vi "Modules DAQ.vi"(8 "error in (no error)":errorcluster) -> (0 "error out":errorcluster)   [LabVIEW 2020]
uses:
  MOTOR/MOTOR.lvlib
  DMM/PalmSens.lvlib
  Hiden Scanner/Hiden Scanner.lvlib
  MRC/MRC Module.lvlib
  WM Pump/Pump.lvlib
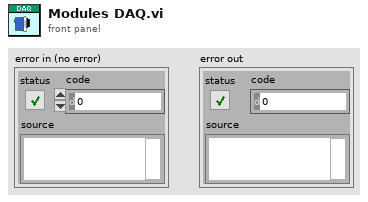
[diagram p1: front panel]
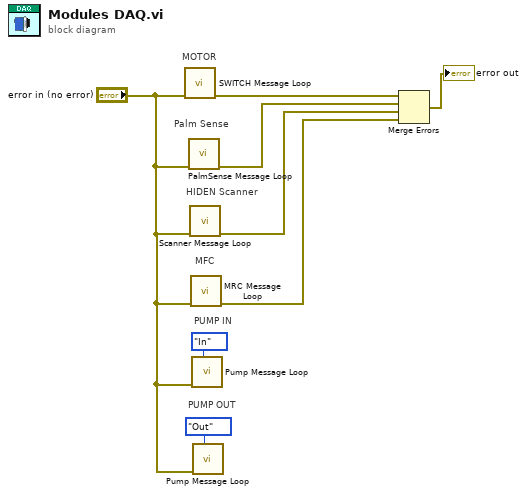
[diagram p0: block diagram]
diagram:
  # "PUMP OUT"
  # "PUMP IN"
  # "MFC"
  # "HIDEN Scanner"
  # "Palm Sense"
  # "MOTOR"
  n1 = call "SWITCH Message Loop.vi"("error in (no error)"="error in (no error)") -> ("error out"=w7:errorcluster)  [unwired: 10 in]
  n2 = call "PalmSense Message Loop.vi"("error in (no error)"="error in (no error)") -> ("error out"=w6:errorcluster)  [unwired: 10 in]
  n3 = call "Scanner Message Loop.vi"("error in (no error)"="error in (no error)") -> ("error out"=w5:errorcluster)  [unwired: 10 in]
  n4 = call "MRC Message Loop.vi"("error in (no error)"="error in (no error)") -> ("error out"=w4:errorcluster)  [unwired: 10 in]
  n5 = call "Pump Message Loop.vi"("Manual Pump Select"=enum32{"In", "Out"}."In", "error in (no error)"="error in (no error)") -> ()  [unwired: 9 in, 1 out]
  n6 = call "Pump Message Loop.vi"("Manual Pump Select"=enum32{"In", "Out"}."Out", "error in (no error)"="error in (no error)") -> ()  [unwired: 9 in, 1 out]
  n7 = Merge Errors(w7, w6, w5, w4) -> (→"error out":errorcluster)
